vi "Get-Set Properties from Cluster.vi"() -> ()   [LabVIEW 2020]
uses:
  Import/_typedefs/frame_parameter_definition.ctl
  Shared/Encoding (Arinc664).ctl
  Scripting/AIM ARINC 664 Scripting.lvlib
  Import/AIM ARINC 664 Import.lvlib
panel:
  in  "Parameter 2":T1 {"encoding" items=["BNR", "BCD", "Discrete", "Signed_32", "Signed_64", "Float_32", "Float_64", "Opaque"]}
  out "error out":errorcluster
  out "data":T3
  out "x = y?":T4
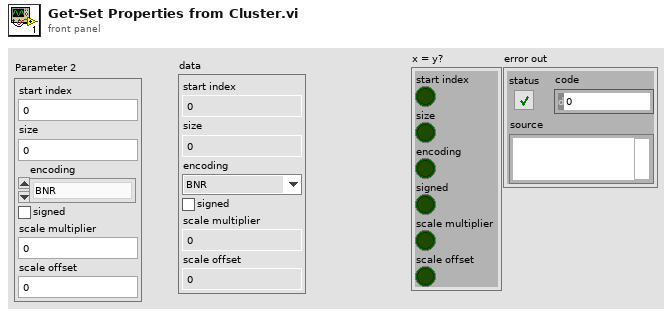
[diagram p1: front panel]
types:
  T1 = typedef "AIM ARINC 664 Import.lvlib/frame_parameter_definition.ctl" = cluster{"start index":i32, "size":i32, "encoding":T2, "signed":bool, "scale multiplier":dbl, "scale offset":dbl}
  T2 = typedef "Encoding (Arinc664).ctl" = u16
  T3 = cluster{"start index":i32, "size":i32, "encoding":enum16{"BNR", "BCD", "Discrete", "Signed_32", "Signed_64", "Float_32", "Float_64", "Opaque"}, "signed":bool, "scale multiplier":dbl, "scale offset":dbl}
  T4 = cluster{"start index":bool, "size":bool, "encoding":bool, "signed":bool, "scale multiplier":bool, "scale offset":bool}
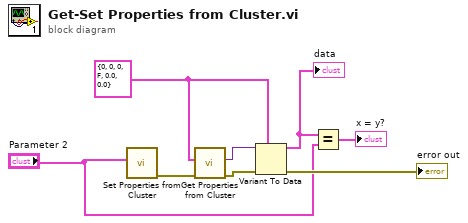
[diagram p0: block diagram]
diagram:
  w1 = T1 {"start index"=0, "size"=0, "encoding"=0, "signed"=FALSE, "scale multiplier"=0.0, "scale offset"=0.0} ("Parameter 2")
  n1 = call "Set Properties from Cluster.vi"("Variant Cluster"="Parameter 2") -> ("error out"=w7:errorcluster)  [unwired: 9 in, 1 out]
  n2 = call "Get Properties from Cluster.vi"("error in"=w7, "Variant Cluster"=w1) -> ("error out"=w4:errorcluster, "data"=w8:variant)  [unwired: 6 in, 2 out]
  n3 = Variant To Data(error in=w4, type=w1, Variant=w8) -> (data=w6:T1, error out=→"error out":errorcluster)
  "data" <- w6
  n4 = Equal?(x=w6, y="Parameter 2") -> (x = y?=→"x = y?":T4)
